vi "refRidders Zero Inner Part.vi"(0 "start/end/f(x)":T2 {"end" format="%.2f"; "start" format="%.2f"; "y value copy" format="%.2f"; "y value" format="%.2f"}, 1 "Variant":variant, 2 "function refnum":T1, 3 "level":dbl, 4 "accuracy":dbl format="%.2f", 5 "case":bool) -> (6 "y value":dbl format="%.2f", 7 "end":dbl format="%.2f", 8 "error":i32)   [LabVIEW 2010, in "NI_Gmath.lvlib"]
uses:
  NI_Gmath.lvlib
  functionRefnum.ctl
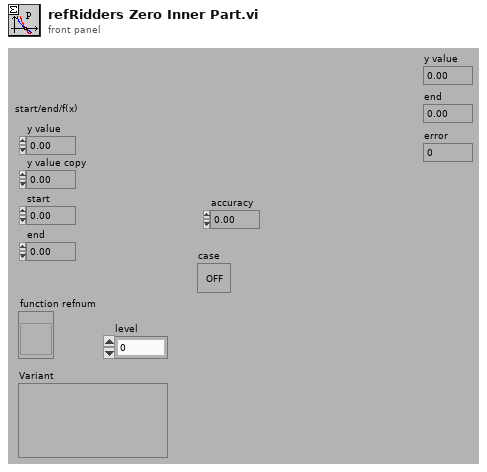
[diagram p1: front panel]
types:
  T1 = typedef "NI_Gmath.lvlib/functionRefnum.ctl" = refnum<vi>
  T2 = cluster{"y value":dbl, "y value copy":dbl, "start":dbl, "end":dbl}
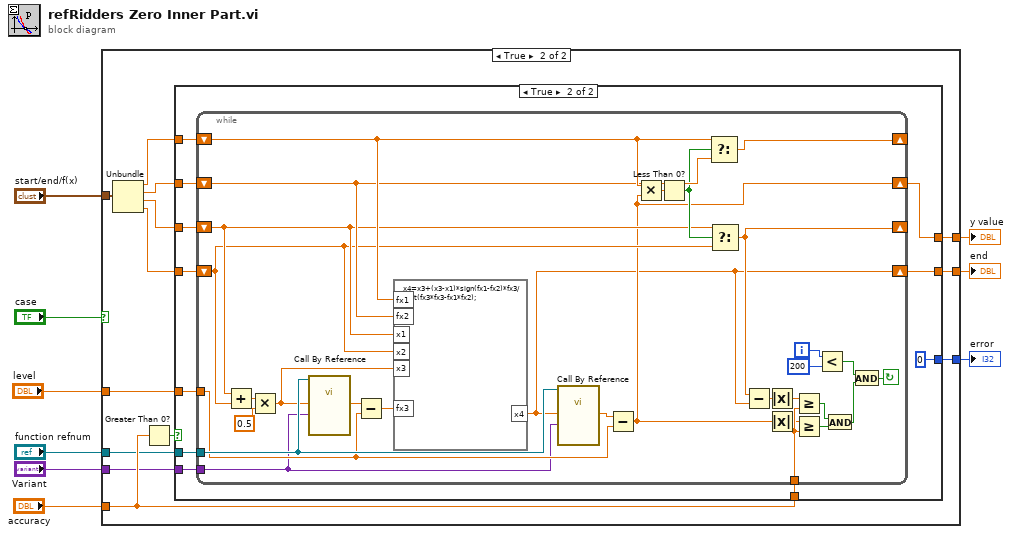
[diagram p0: block diagram]
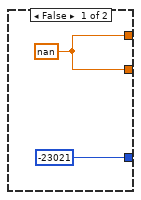
[diagram p2: hidden frame]
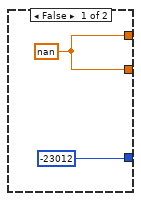
[diagram p3: hidden frame]
diagram:
  n1 = case shown="True" "case" {
    tunnel: [-23021 w23] -> w5
    tunnel: "accuracy" -> [_ w20]
    tunnel: [w10 w22] -> w7
    tunnel: [w10 w21] -> w8
    tunnel: "start/end/f(x)" -> [_ w19]
    tunnel: "function refnum" -> [_ w14]
    tunnel: "Variant" -> [_ w13]
    tunnel: "level" -> [_ w12]
    frame False {
      w10 = nan
    }
    frame True {
      n2 = Unbundle(w19) -> ("y value"=w15:dbl, "y value copy"=w16:dbl, "start"=w17:dbl, "end"=w18:dbl)
      n3 = Greater Than 0?(x=w20) -> (x > 0?=w24:bool)
      n4 = case shown="True" w24 {
        tunnel: w20 -> [_ w37]
        tunnel: w15 -> [_ w36]
        tunnel: w16 -> [_ w35]
        tunnel: w17 -> [_ w34]
        tunnel: w18 -> [_ w33]
        tunnel: [-23012 0] -> w23
        tunnel: [w25 w31] -> w22
        tunnel: [w25 w30] -> w21
        tunnel: w14 -> [_ w29]
        tunnel: w13 -> [_ w28]
        tunnel: w12 -> [_ w27]
        frame False {
          w25 = nan
        }
        frame True {
          n5 = while {
            tunnel: w37 -> [w66]
            shift-left: w35 -> [w50]
            shift-right: [w43] -> w30
            shift-left: w36 -> [w52]
            shift-right: [w51] -> _
            shift-left: w33 -> [w46]
            shift-right: [w38] -> w31
            shift-left: w34 -> [w47]
            shift-right: [w48] -> _
            tunnel: w29 -> [w67]
            tunnel: w28 -> [w39]
            tunnel: w27 -> [w44]
            i -> [w59]
            stop <- w56 continue-if-true
            n6 = Add(x=w47, y=w46) -> (x+y=w64:dbl)
            n7 = Multiply(x=w64, y=0.5) -> (x*y=w41:dbl)
            n8 = call-by-ref "?"(reference=w67, "Variant"=w39, "x"=w41) -> ("f(x)"=w42:dbl)  [unwired: 4 in, 2 out]
            n9 = Subtract(x=w42, y=w44) -> (x-y=w45:dbl)
            n10 = formula code="x4=x3+(x3-x1)*sign(fx1-fx2)*fx3/sqrt(fx3*fx3-fx1*fx2);"("fx1"=w52, "fx2"=w50, "fx3"=w45, "x1"=w47, "x2"=w46, "x3"=w41) -> ("x4"=w38:dbl)
            n11 = call-by-ref "?"(reference=w67, "Variant"=w39, "x"=w38) -> ("f(x)"=w40:dbl)  [unwired: 4 in, 2 out]
            n12 = Subtract(x=w40, y=w44) -> (x-y=w43:dbl)
            n13 = Multiply(x=w52, y=w43) -> (x*y=w63:dbl)
            n14 = Less Than 0?(x=w63) -> (x < 0?=w49:bool)
            n15 = Select(t=w52, s=w49, f=w50) -> (s? t:f=w51:dbl)
            n16 = Select(t=w47, s=w49, f=w46) -> (s? t:f=w48:dbl)
            n17 = Subtract(x=w48, y=w38) -> (x-y=w61:dbl)
            n18 = Absolute Value(x=w61) -> (abs(x)=w62:dbl)
            n19 = Absolute Value(x=w43) -> (abs(x)=w60:dbl)
            n20 = Greater Or Equal?(x=w62, y=w66) -> (x >= y?=w53:bool)
            n21 = Greater Or Equal?(x=w60, y=w66) -> (x >= y?=w54:bool)
            n22 = Less?(x=w59, y=200) -> (x < y?=w57:bool)
            n23 = And(x=w53, y=w54) -> (x .and. y?=w55:bool)
            n24 = And(x=w57, y=w55) -> (x .and. y?=w56:bool)
          }
        }
      }
    }
  }
  "y value" <- w8
  "end" <- w7
  "error" <- w5
